vi "Create Pump.vi"(5 "ConfigManager":refnum<class "ConfigManager.lvclass">, 7 "Shared Resource (F)":bool, 8 "error in (no error)":errorcluster, 10 "Subsystem Name (Pump)":string, 11 "Pump in":refnum<class "Pump.lvclass">) -> (0 "error out":errorcluster, 2 "SMO name":string, 3 "Pump out":refnum<class "Pump.lvclass">)   [LabVIEW 2014, in "Pump.lvclass"]
uses:
  Pump.lvclass
  <vilib>/LabVIEW Open Source Project/Configuration Manager/Manager/ConfigManager.lvclass
  <vilib>/LabVIEW Open Source Project/Configuration Manager/Manager/Decompose KVPs.vi
  <vilib>/LabVIEW Open Source Project/Configuration Manager/Manager/Write.vi
  <vilib>/JKI/JKI SMO/SMO/SMO.lvclass
  <vilib>/LabVIEW Open Source Project/Configuration Manager/Cache/ConfigManager.Cache.lvclass
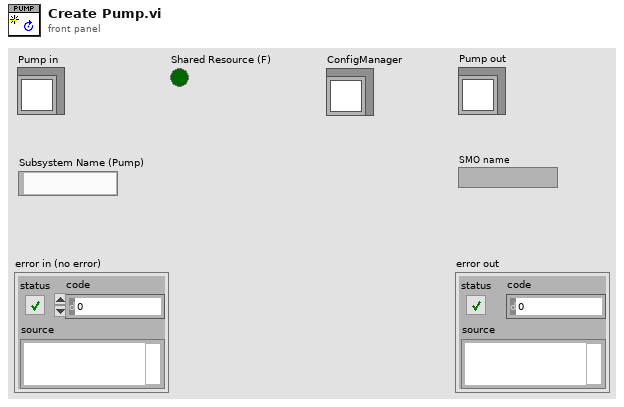
[diagram p1: front panel]
types:
  T1 = typedef "Pump.lvclass/Parameters - cluster.ctl" = cluster{"Kc":dbl, "Ti":dbl, "Td":dbl, "Min Speed":dbl, "Max Speed":dbl}
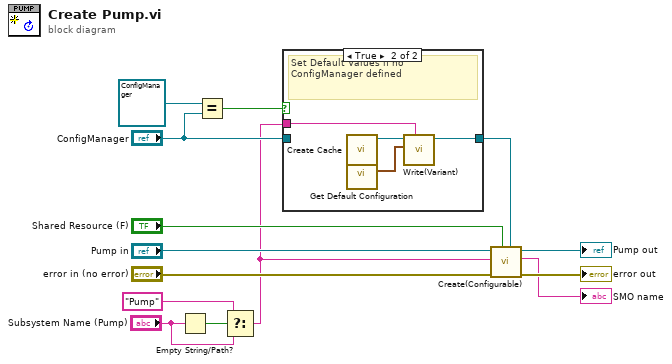
[diagram p0: block diagram]
diagram:
  n1 = Empty String/Path?(string/path="Subsystem Name (Pump)") -> (empty?=w5:bool)
  n2 = Equal?(x=refnum<class "ConfigManager.lvclass"> refnum ("ConfigManager"), y="ConfigManager") -> (x = y?=w1:bool)
  n3 = Select(t="Pump", s=w5, f="Subsystem Name (Pump)") -> (s? t:f=w2:string)
  n4 = case shown="True" w1 {
    tunnel: [w15 w18] -> w10
    tunnel: "ConfigManager" -> [w15 _]
    tunnel: w2 -> [_ w16]
    frame False {
      # "Use Defined ConfigManager"
    }
    frame True {
      # "Set Default Values if no ConfigManager defined"
      n5 = call <vilib>:"Create Cache.vi"() -> ("ConfigManager.Cache"=w19:refnum<class "ConfigManager.Cache.lvclass">)  [unwired: 11 in]
      n6 = call "Get Default Configuration.vi"() -> ("Parameters"=w17:T1)  [unwired: 11 in]
      n7 = call <vilib>:"Write(Variant).vi"("Qualified Name"=w16, "value"=w17, "ConfigManager in"=w19) -> ("ConfigManager out"=w18:refnum<class "ConfigManager.Cache.lvclass">)  [unwired: 6 in, 2 out]
    }
  }
  n8 = call <vilib>:"Create(Configurable).vi"("ConfigManager"=w10, "Shared Resource (F)"="Shared Resource (F)", "error in (no error)"="error in (no error)", "Subsystem Name (optional)"=w2, "SMO"="Pump in") -> ("error out"=→"error out":errorcluster, "SMO name"=→"SMO name":string, "SMO out"=→"Pump out":refnum<class "Pump.lvclass">)  [unwired: 4 in]
